vi "Begin.vi"(11 "Image Size":T1=enum."160x120") -> (0 "error out":errorcluster)   [LabVIEW 2012]
doc: "Called before other user functions, this VI is expected to open initial I/O refnums, load in file data, and do all program initialization. Notice that the <B>error out</B> terminal is simply used for data flow. Wiring it to other structures or subVIs ensures that this VI runs first."
uses:
  <vilib>/Rock Robotics/WPI/Camera/WPI_CameraImageSize.ctl
  <vilib>/Rock Robotics/WPI/DriverStation/WPI_DriverStationRobotMode2.ctl
  <vilib>/Rock Robotics/WPI/Joystick/WPI_JoystickDeviceEnum.ctl
  <vilib>/Rock Robotics/SystemInterfaces/DIO/FPGA_DIOPWMChannel.ctl
  Robot Global Data.vi
  <vilib>/Rock Robotics/WPI/RobotDrive/WPI_RobotDriveOpen2MotorWithJaguar.vi
  <vilib>/Rock Robotics/WPI/Camera/WPI_CameraWhite Balance Values.ctl
  <vilib>/Rock Robotics/WPI/Camera/WPI_CameraExposure Values.ctl
  <vilib>/Rock Robotics/WPI/Camera/WPI_CameraFrameRate.ctl
  <vilib>/Rock Robotics/WPI/SafetyOutput/WPI_SafetyOutputConfigMenu.ctl
  <vilib>/Rock Robotics/SystemInterfaces/DIO/FPGA_DIOChannel.ctl
  <vilib>/Rock Robotics/WPI/Counter/WPI_CounterDigitalInputToDigitalSource.vi
  <vilib>/Rock Robotics/WPI/MotorControl/WPI_MotorControlOpen Victor.vi
  <vilib>/Rock Robotics/WPI/MotorControl/WPI_MotorControlOpenCANJaguar.vi
  <vilib>/Rock Robotics/WPI/CAN/Jaguar/SubVIs/WPI_CANJaguar_ControlMode.ctl
  <vilib>/Rock Robotics/WPI/Solenoid/WPI_SolenoidOpenDouble.vi
  <vilib>/Rock Robotics/WPI/Solenoid/WPI_SolenoidChannel.ctl
  <vilib>/Rock Robotics/SystemInterfaces/Typedef/FPGA_TypedefSolenoidModule.ctl
  <vilib>/Rock Robotics/SystemInterfaces/Typedef/FPGA_TypedefDigitalModule.ctl
  <vilib>/Rock Robotics/SystemInterfaces/DIO/FPGA_DIORelayChannel.ctl
  <vilib>/Rock Robotics/WPI/Solenoid/WPI_SolenoidSetEnum.vi
  <vilib>/Rock Robotics/WPI/Solenoid/WPI_SolenoidValue.ctl
  <vilib>/Rock Robotics/SystemInterfaces/AI/FPGA_AIChannel.ctl
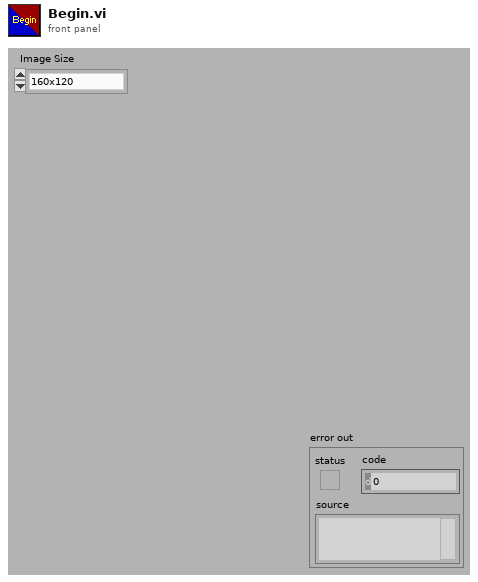
[diagram p1: front panel]
types:
  T1 = typedef "WPI_CameraImageSize.ctl" = enum16{"640x480", "320x240", "160x120"}
  T2 = typedef "FPGA_DIOPWMChannel.ctl" = enum8{"PWM 1", "PWM 2", "PWM 3", "PWM 4", "PWM 5", "PWM 6", "PWM 7", "PWM 8", "PWM 9", "PWM 10", "Invalid"}
  T3 = typedef "WPI_JoystickDeviceEnum.ctl" = enum16{"USB 1", "USB 2", "USB 3", "USB 4", "Kinect 1", "Kinect 2"}
  T4 = typedef "WPI_DriverStationRobotMode2.ctl" = enum16{"Autonomous Disabled", "Autonomous Enabled", "Teleop Disabled", "Teleop Enabled", "Timeout", "Finish", "Test Disabled", "Test Enabled"}
  T5 = typedef "WPI_CameraFrameRate.ctl" = u32
  T6 = typedef "WPI_CameraExposure Values.ctl" = enum16{"Auto", "Flicker-free 50 Hz", "Flicker-free 60 Hz", "Hold current"}
  T7 = typedef "WPI_CameraWhite Balance Values.ctl" = enum16{"Auto", "Fixed indoor", "Fixed outdoor 1", "Fixed outdoor 2", "Fixed fluorescent 1", "Fixed fluorescent 2", "Hold current"}
  T8 = typedef "WPI_CameraDevRef.ctl" = cluster{"Camera Address":string, "CameraStatus":errorcluster, "Acquire Image Notifier":refnum<notifier>}
  T9 = typedef "FPGA_TypedefDigitalModule.ctl" = enum16{"Digital Module 1", "Digital Module 2"}
  T10 = typedef "FPGA_DIORelayChannel.ctl" = enum8{"Relay 1", "Relay 2", "Relay 3", "Relay 4", "Relay 5", "Relay 6", "Relay 7", "Relay 8", "Invalid"}
  T11 = typedef "FPGA_DIOChannel.ctl" = enum8{"DIO 1", "DIO 2", "DIO 3", "DIO 4", "DIO 5", "DIO 6", "DIO 7", "DIO 8", "DIO 9", "DIO 10", "DIO 11", "DIO 12", "DIO 13", "DIO 14", "Invalid"}
  T12 = typedef "WPI_CompressorDevRef.ctl" = cluster{"DevStatus":errorcluster, "DigitalInputDevRef":T13, "RelayDevRef":T14}
  T13 = typedef "WPI_DigitalInputDevRef.ctl" = cluster{"DevStatus":errorcluster, "DIO Channel":T11, "Digital Module":T9}
  T14 = typedef "WPI_RelayDevRef.ctl" = cluster{"DevStatus":errorcluster, "Relay Channel":T10, "Digital Module":T9, "Relay Direction":T15}
  T15 = typedef "WPI_RelayDirection.ctl" = enum16{"Both directions", "Forward only", "Reverse only"}
  T16 = typedef "WPI_SolenoidValue.ctl" = enum16{"Off", "On", "Forward", "Reverse"}
  T17 = typedef "WPI_SolenoidChannel.ctl" = enum8{"Solenoid 1", "Solenoid 2", "Solenoid 3", "Solenoid 4", "Solenoid 5", "Solenoid 6", "Solenoid 7", "Solenoid 8", "Invalid"}
  T18 = typedef "FPGA_TypedefSolenoidModule.ctl" = enum16{"Solenoid Module 1", "Solenoid Module 2"}
  T19 = typedef "WPI_CANJaguar_ControlMode.ctl" = enum8{"Percent VBus", "Current", "Speed", "Position", "Voltage"}
  T20 = typedef "WPI_MotorControlDeviceRef.ctl" = cluster{"DeviceStatus":errorcluster, "Type":enum16{"PWM", "CAN"}, "PWM":cluster{"Digital Module":T9, "PWM Channel":T2, "DeadBand":T21}, "CAN":cluster{"Device Number":u8, "Control Mode":T19, "Semaphore":T22, "Max Vout":dbl}, "Invert":bool, "TransformRef":T23, "InvTransformRef":T23}
  T21 = typedef "WPI_PWMDeadband.ctl" = cluster{"Name":string, "maxPositivePwm":i32, "minPositivePwm":i32, "centerPwm":i32, "maxNegativePwm":i32, "minNegativePwm":i32, "angularRange":u16}
  T22 = typedef "Semaphore RefNum" = refnum<k1>
  T23 = typedef "WPI_PWMTransform_ConPane.ctl" = refnum<vi>
  T24 = typedef "WPI_SolenoidDevRef.ctl" = cluster{"DevStatus":errorcluster, "Solenoid Module":T18, "Forward Solenoid Channel":T17, "Reverse Solenoid Channel":T17}
  T25 = typedef "FPGA_CounterEncoderSourceConvertionLVSourceType.ctl" = cluster{"DevStatus":errorcluster, "AnalogTriggerMode?":bool, "DigitalMode":cluster{"Digital Module":T9, "DIO Channel":T26}, "AnalogTriggerMode":cluster{"AnalogTriggerIndex":T27, "OutputType":T28}}
  T26 = typedef "FPGA_DIODigitalSourceChannel.ctl" = enum8{"DIO 1", "DIO 2", "DIO 3", "DIO 4", "DIO 5", "DIO 6", "DIO 7", "DIO 8", "DIO 9", "DIO 10", "DIO 11", "DIO 12", "DIO 13", "DIO 14", "Disabled"}
  T27 = typedef "FPGA_AnalogTriggerIndex.ctl" = enum8{"Trig 0", "Trig 1", "Trig 2", "Trig 3", "Trig 4", "Trig 5", "Trig 6", "Trig 7", "Invalid"}
  T28 = typedef "FPGA_AnalogTriggerOutType.ctl" = enum16{"InWindow", "TriggerState", "Rising", "Falling"}
  T29 = typedef "WPI_EncoderDevRef.ctl" = cluster{"DevStatus":errorcluster, "EncoderIndex":T30, "CounterIndex":T31, "DistancePerCount":dbl, "Decoding Type":T32}
  T30 = typedef "FPGA_EncoderIdx.ctl" = enum8{"Enc 0", "Enc 1", "Enc 2", "Enc 3", "Invalid"}
  T31 = typedef "FPGA_CounterCtrSystemIndex.ctl" = enum8{"Ctr 0", "Ctr 1", "Ctr 2", "Ctr 3", "Ctr 4", "Ctr 5", "Ctr 6", "Ctr 7", "Invalid"}
  T32 = typedef "WPI_EncoderType.ctl" = enum16{"1x", "2x", "4x"}
  T33 = typedef "WPI_SafetyOutputConfigMenu.ctl" = enum16{"Enable", "Disable"}
  T34 = typedef "WPI_RobotDriveDevRef.ctl" = cluster{"DevStatus":errorcluster, "Motors[]":T20[], "Square Inputs":bool, "Max Output":dbl, "Isochronous":bool}
  T35 = typedef "FPGA_AIChannel.ctl" = enum8{"AI 1", "AI 2", "AI 3", "AI 4", "AI 5", "AI 6", "AI 7", "AI 8", "Invalid"}
  T36 = typedef "WPI_AnalogChannelDevRef.ctl" = cluster{"DevStatus":errorcluster, "Analog Module":T37, "Analog Channel":T35}
  T37 = typedef "FPGA_TypedefAnalogModule.ctl" = enum16{"Analog Module 1", "Analog Module 2"}
  T38 = typedef "WPI_JoystickDevRef.ctl" = cluster{"Device":T3}
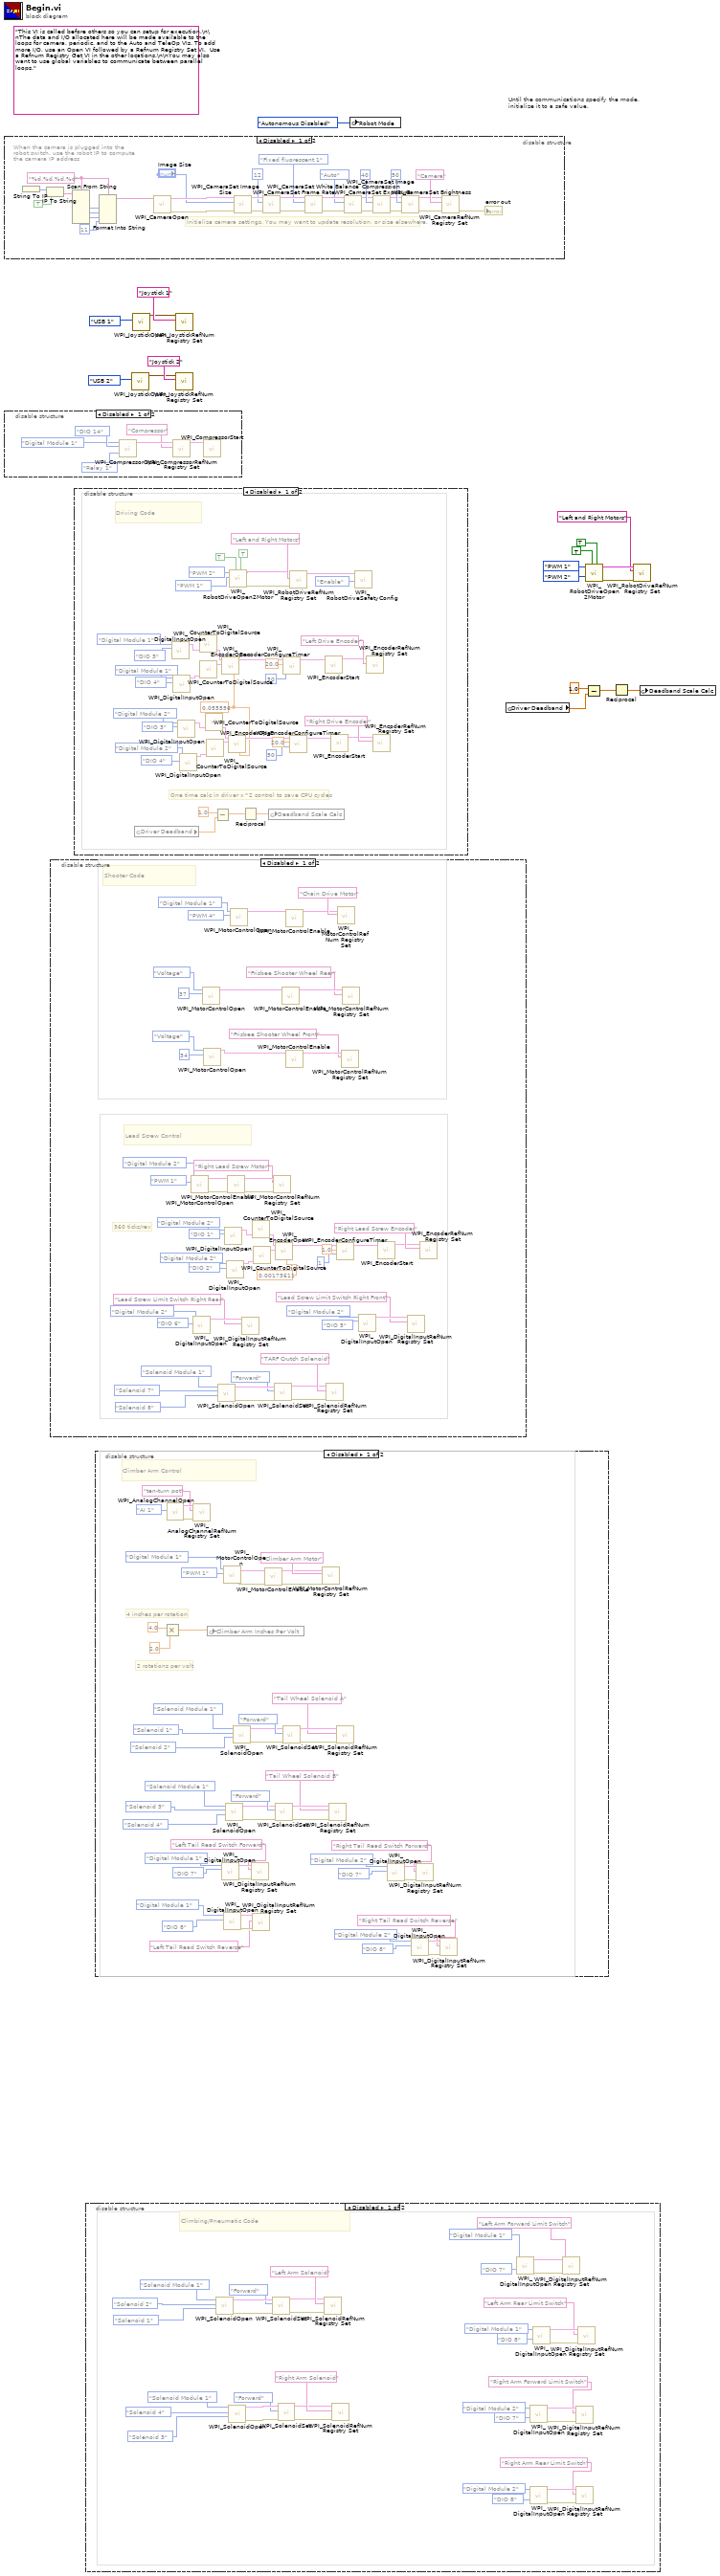
[diagram p0: block diagram]
diagram:
  (unwired) "This VI is called before others so you can setup for execution.\n\nThe data and I/O allocated here will be made available to the loops for camera, periodic, and to the Auto and TeleOp VIs. To add more I/O, use an Open VI followed by a Refnum Registry Set VI.  Use a Refnum Registry Get VI in the other locations.\n\nYou may also want to use global variables to communicate between parallel loops."
  # "Until the communications specify the mode,\ninitialize it to a safe value."
  n1 = disable-structure shown="Disabled" {
    frame Disabled {
      w21 = "%d.%d.%d.%d" ("format string")
      # "When the camera is plugged into the\nrobot switch, use the robot IP to compute\nthe camera IP address"
      # "Initialize camera settings. You may want to update resolution, or size elsewhere."
      n2 = String To IP() -> (0:w28:u32)  [unwired: 1 in]
      n3 = IP To String(1:TRUE ("dot notation? (F)"), 2:w28) -> (0:w26:string)
      n4 = Scan From String(format string=w21, input string=w26) -> (output 1=w25:i32, output 2=w24:i32, output 3=w23:i32)  [unwired: 7 in, 3 out]
      n5 = Format Into String(format string=w21, w25, w24, w23, 11 ("Compression")) -> (resulting string=w20:string)  [unwired: 2 in, 1 out]
      n6 = call <vilib>:"WPI_CameraOpen.vi"("Camera Address"=w20) -> ("error out"=w40:errorcluster, "CameraDevRef"=w41:T8)  [unwired: 1 in, 8 out]
      n7 = call <vilib>:"WPI_CameraSet Image Size.vi"("error in (no error)"=w40, "Image Size"="Image Size", "CameraDevRef"=w41) -> ("error out"=w39:errorcluster, "CameraDevRef Out"=w42:T8)  [unwired: 7 out]
      n8 = call <vilib>:"WPI_CameraSet Frame Rate.vi"("error in (no error)"=w39, "Frame Rate (fps)"=T5 12, "CameraDevRef"=w42) -> ("error out"=w38:errorcluster, "CameraDevRef Out"=w44:T8)  [unwired: 7 out]
      n9 = call <vilib>:"WPI_CameraSet White Balance.vi"("error in (no error)"=w38, "White Balance"=WPI_CameraWhite_Balance_Values."Fixed fluorescent 1", "CameraDevRef"=w44) -> ("error out"=w37:errorcluster, "CameraDevRef Out"=w43:T8)  [unwired: 7 out]
      n10 = call <vilib>:"WPI_CameraSet Exposure.vi"("error in (no error)"=w37, "Exposure"=WPI_CameraExposure_Values."Auto", "CameraDevRef"=w43) -> ("error out"=w36:errorcluster, "CameraDevRef Out"=w46:T8)  [unwired: 7 out]
      n11 = call <vilib>:"WPI_CameraSet Image Compression.vi"("error in (no error)"=w36, "Compression"=40, "CameraDevRef"=w46) -> ("error out"=w35:errorcluster, "CameraDevRef Out"=w45:T8)  [unwired: 7 out]
      n12 = call <vilib>:"WPI_CameraSet Brightness.vi"("error in (no error)"=w35, "Brightness"=50, "CameraDevRef"=w45) -> ("error out"=w33:errorcluster, "CameraDevRef Out"=w34:T8)  [unwired: 7 out]
      n13 = call <vilib>:"WPI_CameraRefNum Registry Set.vi"("error in (no error)"=w33, "refnum name"="Camera", "CameraDevRef"=w34) -> ("error out"=→"error out":errorcluster)  [unwired: 8 out]
    }
    frame Enabled {
    }
  }
  n14 = disable-structure shown="Disabled" {
    frame Disabled {
      n15 = call <vilib>:"WPI_CompressorOpen.vi"("Pressure Switch Digital Module (Module 1)"=FPGA_TypedefDigitalModule."Digital Module 1", "Pressure Switch DIO Channel"=FPGA_DIOChannel."DIO 14", "Relay Channel"=FPGA_DIORelayChannel."Relay 1") -> ("CompressorDevRef"=w53:T12)  [unwired: 11 in, 1 out]
      n16 = call <vilib>:"WPI_CompressorRefNum Registry Set.vi"("refnum name"="Compressor", "CompressorDevRef"=w53) -> ("CompressorDevRef"=w51:T12)  [unwired: 8 in, 1 out]
      n17 = call <vilib>:"WPI_CompressorStart.vi"("CompressorDevRef"=w51) -> ()  [unwired: 9 in, 2 out]
    }
    frame Enabled {
    }
  }
  n18 = disable-structure shown="Disabled" {
    frame Disabled {
      # "Lead Screw Control"
      # "Shooter Code"
      # "360 ticks/rev"
      n19 = call-poly <vilib>:"WPI_MotorControlOpen.vi"("PWM Channel"=FPGA_DIOPWMChannel."PWM 1", "Digital Module (Module 1)"=FPGA_TypedefDigitalModule."Digital Module 2") -> ("error out"=w108:errorcluster, "MotorControlDeviceRef"=w107:T20)  [unwired: 8 in]
      n20 = call <vilib>:"WPI_DigitalInputOpen.vi"("DIO Channel"=FPGA_DIOChannel."DIO 6", "Digital Module (Module 1)"=FPGA_TypedefDigitalModule."Digital Module 2") -> ("DigitalInputDevRef"=w91:T13)  [unwired: 8 in, 1 out]
      n21 = call-poly <vilib>:"WPI_MotorControlOpen.vi"("Device Number"=u8 37, "Control Mode"=WPI_CANJaguar_ControlMode."Voltage") -> ("MotorControlDeviceRef"=w75:T20)  [unwired: 8 in, 1 out]
      n22 = call-poly <vilib>:"WPI_MotorControlOpen.vi"("Device Number"=u8 34, "Control Mode"=WPI_CANJaguar_ControlMode."Voltage") -> ("MotorControlDeviceRef"=w74:T20)  [unwired: 8 in, 1 out]
      n23 = call-poly <vilib>:"WPI_SolenoidOpen.vi"("Reverse Solenoid Channel"=WPI_SolenoidChannel."Solenoid 8", "Forward Solenoid Channel"=WPI_SolenoidChannel."Solenoid 7", "Solenoid Module (Module 1)"=FPGA_TypedefSolenoidModule."Solenoid Module 1") -> ("error out"=w60:errorcluster, "SolenoidDevRef"=w59:T24)  [unwired: 7 in]
      n24 = call <vilib>:"WPI_DigitalInputOpen.vi"("DIO Channel"=FPGA_DIOChannel."DIO 1", "Digital Module (Module 1)"=FPGA_TypedefDigitalModule."Digital Module 2") -> ("DigitalInputDevRef"=w66:T13)  [unwired: 8 in, 1 out]
      n25 = call <vilib>:"WPI_DigitalInputOpen.vi"("DIO Channel"=FPGA_DIOChannel."DIO 2", "Digital Module (Module 1)"=FPGA_TypedefDigitalModule."Digital Module 2") -> ("DigitalInputDevRef"=w65:T13)  [unwired: 8 in, 1 out]
      n26 = call <vilib>:"WPI_MotorControlEnable.vi"("error in (no error)"=w108, "CAN Jaguar Ref"=w107) -> ("error out"=w106:errorcluster, "CAN Jaguar Ref Out"=w105:T20)  [unwired: 8 in]
      n27 = call-poly <vilib>:"WPI_MotorControlOpen.vi"("PWM Channel"=FPGA_DIOPWMChannel."PWM 4", "Digital Module (Module 1)"=FPGA_TypedefDigitalModule."Digital Module 1") -> ("MotorControlDeviceRef"=w79:T20)  [unwired: 8 in, 1 out]
      n28 = call <vilib>:"WPI_DigitalInputRefNum Registry Set.vi"("refnum name"="Lead Screw Limit Switch Right Rear", "DigitalInputDevRef"=w91) -> ()  [unwired: 8 in, 2 out]
      n29 = call-poly <vilib>:"WPI_CounterToDigitalSource.vi"("DigitalInputDevRef"=w66) -> ("Digital Source"=w98:T25)  [unwired: 6 in]
      n30 = call-poly <vilib>:"WPI_CounterToDigitalSource.vi"("DigitalInputDevRef"=w65) -> ("Digital Source"=w99:T25)  [unwired: 6 in]
      n31 = call <vilib>:"WPI_MotorControlRefNum Registry Set.vi"("error in (no error)"=w106, "refnum name"="Right Lead Screw Motor", "MotorControlDevRef"=w105) -> ()  [unwired: 7 in, 2 out]
      n32 = call-poly <vilib>:"WPI_SolenoidSet.vi"("error in (no error)"=w60, "Value"=WPI_SolenoidValue."Forward", "SolenoidDevRef"=w59) -> ("error out"=w57:errorcluster, "SolenoidDevRef"=w58:T24)  [unwired: 7 in]
      n33 = call <vilib>:"WPI_EncoderOpen.vi"("DistancePerCount"=0.00173611 ("Distance Per Line(in.)"), "BSource"=w99, "ASource"=w98) -> ("EncoderDevRef"=w100:T29)  [unwired: 7 in, 1 out]
      n34 = call <vilib>:"WPI_MotorControlEnable.vi"("CAN Jaguar Ref"=w75) -> ("CAN Jaguar Ref Out"=w73:T20)  [unwired: 9 in, 1 out]
      n35 = call <vilib>:"WPI_MotorControlEnable.vi"("CAN Jaguar Ref"=w79) -> ("CAN Jaguar Ref Out"=w78:T20)  [unwired: 9 in, 1 out]
      n36 = call <vilib>:"WPI_MotorControlEnable.vi"("CAN Jaguar Ref"=w74) -> ("CAN Jaguar Ref Out"=w72:T20)  [unwired: 9 in, 1 out]
      n37 = call <vilib>:"WPI_SolenoidRefNum Registry Set.vi"("error in (no error)"=w57, "refnum name"="TARF Crutch Solenoid", "SolenoidDevRef"=w58) -> ()  [unwired: 7 in, 2 out]
      n38 = call <vilib>:"WPI_EncoderConfigureTimer.vi"("Number Samples to Average"=u8 1, "Minimum Rate"=1.0, "EncoderDevRef"=w100) -> ("EncoderDevRef"=w101:T29)  [unwired: 7 in, 1 out]
      n39 = call <vilib>:"WPI_MotorControlRefNum Registry Set.vi"("refnum name"="Chain Drive Motor", "MotorControlDevRef"=w78) -> ()  [unwired: 8 in, 2 out]
      n40 = call <vilib>:"WPI_MotorControlRefNum Registry Set.vi"("refnum name"="Frisbee Shooter Wheel Front", "MotorControlDevRef"=w72) -> ()  [unwired: 8 in, 2 out]
      n41 = call <vilib>:"WPI_MotorControlRefNum Registry Set.vi"("refnum name"="Frisbee Shooter Wheel Rear", "MotorControlDevRef"=w73) -> ()  [unwired: 8 in, 2 out]
      n42 = call <vilib>:"WPI_DigitalInputOpen.vi"("DIO Channel"=FPGA_DIOChannel."DIO 5", "Digital Module (Module 1)"=FPGA_TypedefDigitalModule."Digital Module 2") -> ("DigitalInputDevRef"=w88:T13)  [unwired: 8 in, 1 out]
      n43 = call <vilib>:"WPI_EncoderStart.vi"("EncoderDevRef"=w101) -> ("EncoderDevRef"=w102:T29)  [unwired: 9 in, 1 out]
      n44 = call <vilib>:"WPI_DigitalInputRefNum Registry Set.vi"("refnum name"="Lead Screw Limit Switch Right Front", "DigitalInputDevRef"=w88) -> ()  [unwired: 8 in, 2 out]
      n45 = call <vilib>:"WPI_EncoderRefNum Registry Set.vi"("refnum name"="Right Lead Screw Encoder", "EncoderDevRef"=w102) -> ()  [unwired: 8 in, 2 out]
    }
    frame Enabled {
    }
  }
  n46 = disable-structure shown="Disabled" {
    frame Disabled {
      w120 = 0.055556 ("Distance Per Line(in.)")
      # "Driving Code"
      # "One time calc in driver x^2 control to save CPU cycles"
      n47 = global read "Robot Global Data.vi" "Driver Deadband"() -> (w147:dbl)
      n48 = call <vilib>:"WPI_DigitalInputOpen.vi"("DIO Channel"=FPGA_DIOChannel."DIO 3", "Digital Module (Module 1)"=FPGA_TypedefDigitalModule."Digital Module 1") -> ("DigitalInputDevRef"=w127:T13)  [unwired: 8 in, 1 out]
      n49 = call <vilib>:"WPI_DigitalInputOpen.vi"("DIO Channel"=FPGA_DIOChannel."DIO 4", "Digital Module (Module 1)"=FPGA_TypedefDigitalModule."Digital Module 1") -> ("DigitalInputDevRef"=w129:T13)  [unwired: 8 in, 1 out]
      n50 = call <vilib>:"WPI_DigitalInputOpen.vi"("DIO Channel"=FPGA_DIOChannel."DIO 3", "Digital Module (Module 1)"=FPGA_TypedefDigitalModule."Digital Module 2") -> ("DigitalInputDevRef"=w137:T13)  [unwired: 8 in, 1 out]
      n51 = call <vilib>:"WPI_DigitalInputOpen.vi"("DIO Channel"=FPGA_DIOChannel."DIO 4", "Digital Module (Module 1)"=FPGA_TypedefDigitalModule."Digital Module 2") -> ("DigitalInputDevRef"=w139:T13)  [unwired: 8 in, 1 out]
      n52 = call-poly <vilib>:"WPI_CounterToDigitalSource.vi"("DigitalInputDevRef"=w127) -> ("Digital Source"=w128:T25)  [unwired: 6 in]
      n53 = call-poly <vilib>:"WPI_CounterToDigitalSource.vi"("DigitalInputDevRef"=w129) -> ("Digital Source"=w130:T25)  [unwired: 6 in]
      n54 = call-poly <vilib>:"WPI_CounterToDigitalSource.vi"("DigitalInputDevRef"=w137) -> ("Digital Source"=w138:T25)  [unwired: 6 in]
      n55 = call-poly <vilib>:"WPI_CounterToDigitalSource.vi"("DigitalInputDevRef"=w139) -> ("Digital Source"=w140:T25)  [unwired: 6 in]
      n56 = Subtract(x=1.0, y=w147) -> (x-y=w146:dbl)
      n57 = call <vilib>:"WPI_EncoderOpen.vi"("DistancePerCount"=w120, "BSource"=w130, "ASource"=w128) -> ("EncoderDevRef"=w131:T29)  [unwired: 7 in, 1 out]
      n58 = call <vilib>:"WPI_EncoderOpen.vi"("DistancePerCount"=w120, "BSource"=w140, "ASource"=w138) -> ("EncoderDevRef"=w141:T29)  [unwired: 7 in, 1 out]
      n59 = call-poly <vilib>:"WPI_RobotDriveOpen2Motor.vi"("Right Motor Inverted"=TRUE, "Left Motor Inverted"=TRUE, "Right Motor"=FPGA_DIOPWMChannel."PWM 1", "Left Motor"=FPGA_DIOPWMChannel."PWM 2") -> ("error out"=w114:errorcluster, "RobotDriveDevRef"=w115:T34)  [unwired: 6 in]
      n60 = Reciprocal(x=w146) -> (1/x=w145:dbl)
      n61 = global write "Robot Global Data.vi" "Deadband Scale Calc"(w145) -> ()
      n62 = call <vilib>:"WPI_EncoderConfigureTimer.vi"("Number Samples to Average"=u8 50, "Minimum Rate"=20.0, "EncoderDevRef"=w131) -> ("EncoderDevRef"=w132:T29)  [unwired: 7 in, 1 out]
      n63 = call <vilib>:"WPI_EncoderConfigureTimer.vi"("Number Samples to Average"=u8 50, "Minimum Rate"=20.0, "EncoderDevRef"=w141) -> ("EncoderDevRef"=w142:T29)  [unwired: 7 in, 1 out]
      n64 = call <vilib>:"WPI_RobotDriveRefNum Registry Set.vi"("error in (no error)"=w114, "refnum name"="Left and Right Motors", "RobotDriveDevRef"=w115) -> ("RobotDriveDevRef"=w150:T34)  [unwired: 8 out]
      n65 = call <vilib>:"WPI_EncoderStart.vi"("EncoderDevRef"=w132) -> ("EncoderDevRef"=w133:T29)  [unwired: 9 in, 1 out]
      n66 = call <vilib>:"WPI_EncoderStart.vi"("EncoderDevRef"=w142) -> ("EncoderDevRef"=w143:T29)  [unwired: 9 in, 1 out]
      n67 = call <vilib>:"WPI_RobotDriveSafetyConfig.vi"("mode"=WPI_SafetyOutputConfigMenu."Enable", "RobotDriveDevRef"=w150) -> ()  [unwired: 8 in, 2 out]
      n68 = call <vilib>:"WPI_EncoderRefNum Registry Set.vi"("refnum name"="Left Drive Encoder", "EncoderDevRef"=w133) -> ()  [unwired: 8 in, 2 out]
      n69 = call <vilib>:"WPI_EncoderRefNum Registry Set.vi"("refnum name"="Right Drive Encoder", "EncoderDevRef"=w143) -> ()  [unwired: 8 in, 2 out]
    }
    frame Enabled {
    }
  }
  n70 = disable-structure shown="Disabled" {
    frame Disabled {
      # "Climbing/Pneumatic Code"
      n71 = call-poly <vilib>:"WPI_SolenoidOpen.vi"("Reverse Solenoid Channel"=WPI_SolenoidChannel."Solenoid 1", "Forward Solenoid Channel"=WPI_SolenoidChannel."Solenoid 2", "Solenoid Module (Module 1)"=FPGA_TypedefSolenoidModule."Solenoid Module 1") -> ("error out"=w161:errorcluster, "SolenoidDevRef"=w160:T24)  [unwired: 7 in]
      n72 = call-poly <vilib>:"WPI_SolenoidOpen.vi"("Reverse Solenoid Channel"=WPI_SolenoidChannel."Solenoid 3", "Forward Solenoid Channel"=WPI_SolenoidChannel."Solenoid 4", "Solenoid Module (Module 1)"=FPGA_TypedefSolenoidModule."Solenoid Module 1") -> ("error out"=w158:errorcluster, "SolenoidDevRef"=w159:T24)  [unwired: 7 in]
      n73 = call-poly <vilib>:"WPI_SolenoidSet.vi"("error in (no error)"=w161, "Value"=WPI_SolenoidValue."Forward", "SolenoidDevRef"=w160) -> ("error out"=w156:errorcluster, "SolenoidDevRef"=w157:T24)  [unwired: 7 in]
      n74 = call-poly <vilib>:"WPI_SolenoidSet.vi"("error in (no error)"=w158, "Value"=WPI_SolenoidValue."Forward", "SolenoidDevRef"=w159) -> ("error out"=w154:errorcluster, "SolenoidDevRef"=w155:T24)  [unwired: 7 in]
      n75 = call <vilib>:"WPI_SolenoidRefNum Registry Set.vi"("error in (no error)"=w156, "refnum name"="Left Arm Solenoid", "SolenoidDevRef"=w157) -> ()  [unwired: 7 in, 2 out]
      n76 = call <vilib>:"WPI_SolenoidRefNum Registry Set.vi"("error in (no error)"=w154, "refnum name"="Right Arm Solenoid", "SolenoidDevRef"=w155) -> ()  [unwired: 7 in, 2 out]
      n77 = call <vilib>:"WPI_DigitalInputOpen.vi"("DIO Channel"=FPGA_DIOChannel."DIO 7", "Digital Module (Module 1)"=FPGA_TypedefDigitalModule."Digital Module 1") -> ("error out"=w178:errorcluster, "DigitalInputDevRef"=w179:T13)  [unwired: 8 in]
      n78 = call <vilib>:"WPI_DigitalInputOpen.vi"("DIO Channel"=FPGA_DIOChannel."DIO 7", "Digital Module (Module 1)"=FPGA_TypedefDigitalModule."Digital Module 2") -> ("error out"=w168:errorcluster, "DigitalInputDevRef"=w169:T13)  [unwired: 8 in]
      n79 = call <vilib>:"WPI_DigitalInputOpen.vi"("DIO Channel"=FPGA_DIOChannel."DIO 8", "Digital Module (Module 1)"=FPGA_TypedefDigitalModule."Digital Module 2") -> ("error out"=w164:errorcluster, "DigitalInputDevRef"=w165:T13)  [unwired: 8 in]
      n80 = call <vilib>:"WPI_DigitalInputOpen.vi"("DIO Channel"=FPGA_DIOChannel."DIO 8", "Digital Module (Module 1)"=FPGA_TypedefDigitalModule."Digital Module 1") -> ("error out"=w173:errorcluster, "DigitalInputDevRef"=w174:T13)  [unwired: 8 in]
      n81 = call <vilib>:"WPI_DigitalInputRefNum Registry Set.vi"("error in (no error)"=w178, "refnum name"="Left Arm Forward Limit Switch", "DigitalInputDevRef"=w179) -> ()  [unwired: 7 in, 2 out]
      n82 = call <vilib>:"WPI_DigitalInputRefNum Registry Set.vi"("error in (no error)"=w168, "refnum name"="Right Arm Forward Limit Switch", "DigitalInputDevRef"=w169) -> ()  [unwired: 7 in, 2 out]
      n83 = call <vilib>:"WPI_DigitalInputRefNum Registry Set.vi"("error in (no error)"=w164, "refnum name"="Right Arm Rear Limit Switch", "DigitalInputDevRef"=w165) -> ()  [unwired: 7 in, 2 out]
      n84 = call <vilib>:"WPI_DigitalInputRefNum Registry Set.vi"("error in (no error)"=w173, "refnum name"="Left Arm Rear Limit Switch", "DigitalInputDevRef"=w174) -> ()  [unwired: 7 in, 2 out]
    }
    frame Enabled {
    }
  }
  n85 = disable-structure shown="Disabled" {
    frame Disabled {
      # "2 rotations per volt"
      # "4 inches per rotation"
      # "Climber Arm Control"
      n86 = Multiply(x=4.0, y=2.0) -> (x*y=w232:dbl)
      n87 = call <vilib>:"WPI_AnalogChannelOpen.vi"("Analog Channel"=FPGA_AIChannel."AI 1") -> ("error out"=w240:errorcluster, "AIDeviceRef"=w239:T36)  [unwired: 9 in]
      n88 = call <vilib>:"WPI_AnalogChannelRefNum Registry Set.vi"("error in (no error)"=w240, "refnum name"="ten-turn pot", "AIDeviceRef"=w239) -> ()  [unwired: 7 in, 2 out]
      n89 = global write "Robot Global Data.vi" "Climber Arm Inches Per Volt"(w232) -> ()
      n90 = call <vilib>:"WPI_DigitalInputOpen.vi"("DIO Channel"=FPGA_DIOChannel."DIO 7", "Digital Module (Module 1)"=FPGA_TypedefDigitalModule."Digital Module 1") -> ("error out"=w209:errorcluster, "DigitalInputDevRef"=w208:T13)  [unwired: 8 in]
      n91 = call-poly <vilib>:"WPI_MotorControlOpen.vi"("PWM Channel"=FPGA_DIOPWMChannel."PWM 1", "Digital Module (Module 1)"=FPGA_TypedefDigitalModule."Digital Module 1") -> ("error out"=w212:errorcluster, "MotorControlDeviceRef"=w213:T20)  [unwired: 8 in]
      n92 = call <vilib>:"WPI_DigitalInputOpen.vi"("DIO Channel"=FPGA_DIOChannel."DIO 8", "Digital Module (Module 1)"=FPGA_TypedefDigitalModule."Digital Module 1") -> ("error out"=w206:errorcluster, "DigitalInputDevRef"=w207:T13)  [unwired: 8 in]
      n93 = call-poly <vilib>:"WPI_SolenoidOpen.vi"("Reverse Solenoid Channel"=WPI_SolenoidChannel."Solenoid 4", "Forward Solenoid Channel"=WPI_SolenoidChannel."Solenoid 3", "Solenoid Module (Module 1)"=FPGA_TypedefSolenoidModule."Solenoid Module 1") -> ("error out"=w218:errorcluster, "SolenoidDevRef"=w217:T24)  [unwired: 7 in]
      n94 = call-poly <vilib>:"WPI_SolenoidOpen.vi"("Reverse Solenoid Channel"=WPI_SolenoidChannel."Solenoid 2", "Forward Solenoid Channel"=WPI_SolenoidChannel."Solenoid 1", "Solenoid Module (Module 1)"=FPGA_TypedefSolenoidModule."Solenoid Module 1") -> ("error out"=w227:errorcluster, "SolenoidDevRef"=w226:T24)  [unwired: 7 in]
      n95 = call <vilib>:"WPI_DigitalInputRefNum Registry Set.vi"("error in (no error)"=w209, "refnum name"="Left Tail Read Switch Forward", "DigitalInputDevRef"=w208) -> ()  [unwired: 7 in, 2 out]
      n96 = call <vilib>:"WPI_DigitalInputRefNum Registry Set.vi"("error in (no error)"=w206, "refnum name"="Left Tail Read Switch Reverse", "DigitalInputDevRef"=w207) -> ()  [unwired: 7 in, 2 out]
      n97 = call <vilib>:"WPI_MotorControlEnable.vi"("error in (no error)"=w212, "CAN Jaguar Ref"=w213) -> ("error out"=w210:errorcluster, "CAN Jaguar Ref Out"=w211:T20)  [unwired: 8 in]
      n98 = call-poly <vilib>:"WPI_SolenoidSet.vi"("error in (no error)"=w218, "Value"=WPI_SolenoidValue."Forward", "SolenoidDevRef"=w217) -> ("error out"=w220:errorcluster, "SolenoidDevRef"=w219:T24)  [unwired: 7 in]
      n99 = call-poly <vilib>:"WPI_SolenoidSet.vi"("error in (no error)"=w227, "Value"=WPI_SolenoidValue."Forward", "SolenoidDevRef"=w226) -> ("error out"=w229:errorcluster, "SolenoidDevRef"=w228:T24)  [unwired: 7 in]
      n100 = call <vilib>:"WPI_MotorControlRefNum Registry Set.vi"("error in (no error)"=w210, "refnum name"="Climber Arm Motor", "MotorControlDevRef"=w211) -> ()  [unwired: 7 in, 2 out]
      n101 = call <vilib>:"WPI_SolenoidRefNum Registry Set.vi"("error in (no error)"=w220, "refnum name"="Tail Wheel Solenoid B", "SolenoidDevRef"=w219) -> ()  [unwired: 7 in, 2 out]
      n102 = call <vilib>:"WPI_SolenoidRefNum Registry Set.vi"("error in (no error)"=w229, "refnum name"="Tail Wheel Solenoid A", "SolenoidDevRef"=w228) -> ()  [unwired: 7 in, 2 out]
      n103 = call <vilib>:"WPI_DigitalInputOpen.vi"("DIO Channel"=FPGA_DIOChannel."DIO 7", "Digital Module (Module 1)"=FPGA_TypedefDigitalModule."Digital Module 2") -> ("error out"=w199:errorcluster, "DigitalInputDevRef"=w198:T13)  [unwired: 8 in]
      n104 = call <vilib>:"WPI_DigitalInputOpen.vi"("DIO Channel"=FPGA_DIOChannel."DIO 8", "Digital Module (Module 1)"=FPGA_TypedefDigitalModule."Digital Module 2") -> ("error out"=w194:errorcluster, "DigitalInputDevRef"=w193:T13)  [unwired: 8 in]
      n105 = call <vilib>:"WPI_DigitalInputRefNum Registry Set.vi"("error in (no error)"=w199, "refnum name"="Right Tail Read Switch Forward", "DigitalInputDevRef"=w198) -> ()  [unwired: 7 in, 2 out]
      n106 = call <vilib>:"WPI_DigitalInputRefNum Registry Set.vi"("error in (no error)"=w194, "refnum name"="Right Tail Read Switch Reverse", "DigitalInputDevRef"=w193) -> ()  [unwired: 7 in, 2 out]
    }
    frame Enabled {
    }
  }
  n107 = call <vilib>:"WPI_JoystickOpen.vi"("JoystickDevice"=WPI_JoystickDeviceEnum."USB 2") -> ("JoystickDevRef"=w13:T38)  [unwired: 10 in]
  n108 = call <vilib>:"WPI_JoystickOpen.vi"("JoystickDevice"=WPI_JoystickDeviceEnum."USB 1") -> ("JoystickDevRef"=w16:T38)  [unwired: 10 in]
  n109 = call <vilib>:"WPI_JoystickRefNum Registry Set.vi"("refnum name"="Joystick 2", "JoystickDevRef"=w13) -> ()  [unwired: 8 in, 2 out]
  n110 = call <vilib>:"WPI_JoystickRefNum Registry Set.vi"("refnum name"="Joystick 1", "JoystickDevRef"=w16) -> ()  [unwired: 8 in, 2 out]
  n111 = global write "Robot Global Data.vi" "Robot Mode"(WPI_DriverStationRobotMode2."Autonomous Disabled" ("Robot Mode")) -> ()
  n112 = global read "Robot Global Data.vi" "Driver Deadband"() -> (w5:dbl)
  n113 = Subtract(x=1.0, y=w5) -> (x-y=w4:dbl)
  n114 = call-poly <vilib>:"WPI_RobotDriveOpen2Motor.vi"("Right Motor Inverted"=TRUE, "Left Motor Inverted"=TRUE, "Right Motor"=FPGA_DIOPWMChannel."PWM 2", "Left Motor"=FPGA_DIOPWMChannel."PWM 1") -> ("error out"=w9:errorcluster, "RobotDriveDevRef"=w8:T34)  [unwired: 6 in]
  n115 = Reciprocal(x=w4) -> (1/x=w3:dbl)
  n116 = call <vilib>:"WPI_RobotDriveRefNum Registry Set.vi"("error in (no error)"=w9, "refnum name"="Left and Right Motors", "RobotDriveDevRef"=w8) -> ()  [unwired: 7 in, 2 out]
  n117 = global write "Robot Global Data.vi" "Deadband Scale Calc"(w3) -> ()
